vi "PAINEL DE TESTES 2808.vi"() -> ()   [LabVIEW 2019]
panel:
  in  "stop":bool
  out "ADDR NÃO COMPATÍVEL":bool
  in  "ME":bool
  in  "HMP":bool
  in  "SMP":bool
  out "TAM_P":bool
  out "POS_1":bool
  out "MAT":bool
  out "POS_2":bool
  out "COR_3":bool
  out "PDS":bool
  out "COR_2":bool
  out "PEE":bool
  out "POS_4":bool
  out "COR_1":bool
  out "POS_3":bool
  out "TAM_M":bool
  out "TAM_G":bool
  out "ADDR 100":bool
  out "ADDR 101":bool
  out "ADDR 011":bool
  out "ADDR 010":bool
  in  "ADDR ARRAY":bool[](array[boolean])
  out "INPUT ARRAYS":bool[](array[boolean])
  in  "time stamp":timestamp format="%<%X\n%x>T"
  # "UNIVERSIDADE FEDERAL DE SÃO JOÃO DEL-REI"
  # "CAMPUS ALTO PARAOPEBA - ENGENHARIA MECATRÔNICA\nLABORATÓRIO DE CONTROLE E AUTOMAÇÃO"
  # "PAINEL DE TESTES DO MÓDULO 2808"
  # "P1.0"
  # "P1.1"
  # "P1.2"
  # "D0"
  # "D1"
  # "D2"
  # "D3"
  # "D4"
  # "D5"
  # "D6"
  # "D7"
  # "ADDR 010"
  # "TAGS:\nPEE - PEÇA NA ENTRADA DA ESTEIRA\nMAT - MATERIAL DA PEÇA (T=METAL)\nCOR_1 - PEÇA DA COR 1\nCOR_2 - PEÇA DA COR 2\nCOR_3 - PEÇA DA COR 3\nTAM_G - PEÇA GRANDE\nTAM_M - PEÇA MÉDIA\nTAM_P - PEÇA PEQUENA\nPOS_1 - HASTE NA POSIÇÃO 1\nPOS_2 - HASTE NA POSIÇÃO 2\nPOS_3 - HASTE NA POSIÇÃO 3\nPOS_4 - HASTE NA POSIÇÃO 4\nPDS - PEÇA DEPOSITADA NO SLOT\n\nSMP - SENTIDO DO MOTOR DE PASSO\nHMP - HABILITA MOTOR DE PASSO\nME - MOTOR ESTEIRA"
  # "ADDR 011"
  # "ENCODER"
  # "ADDR 101"
  # "ADDR 100"
  # "TAM_G"
  # "TAM_P"
  # "TAM_M"
  # "SMP"
  # "POS_1"
  # "POS_2"
  # "POS_3"
  # "POS_4"
  # "PEE"
  # "MAT"
  # "COR_1,2,3"
  # "HMP"
  # "ME"
  # "PDS"
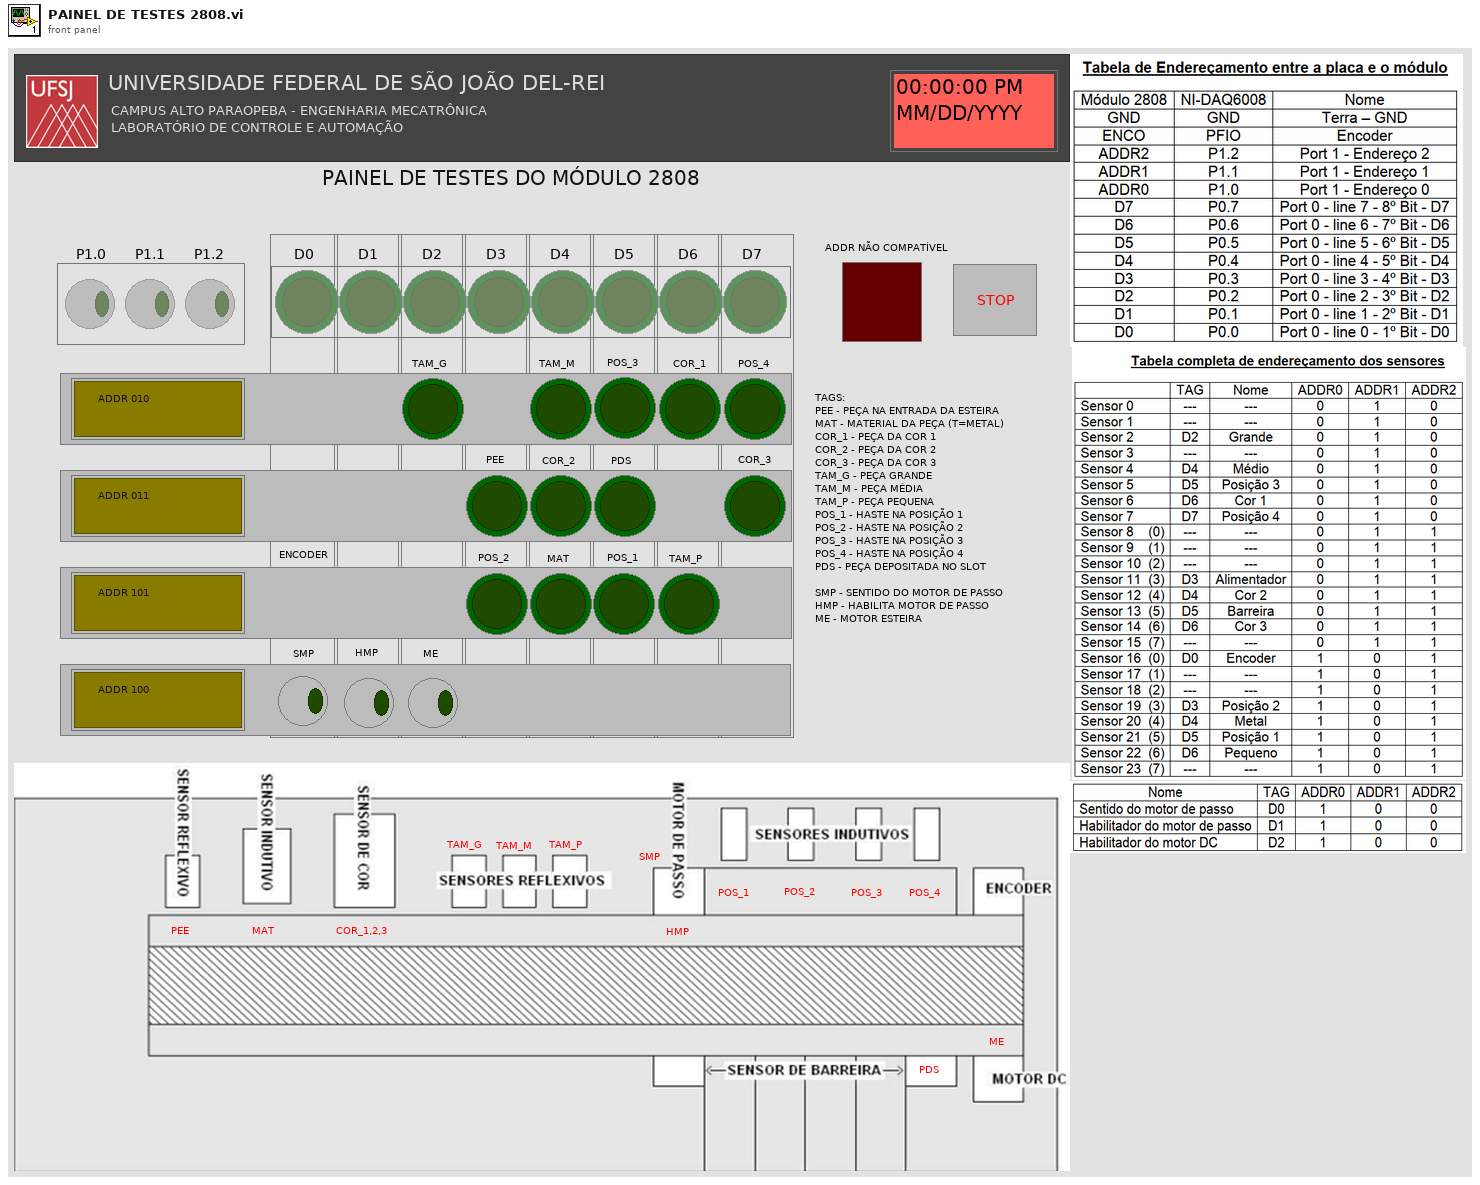
[diagram p1: front panel]
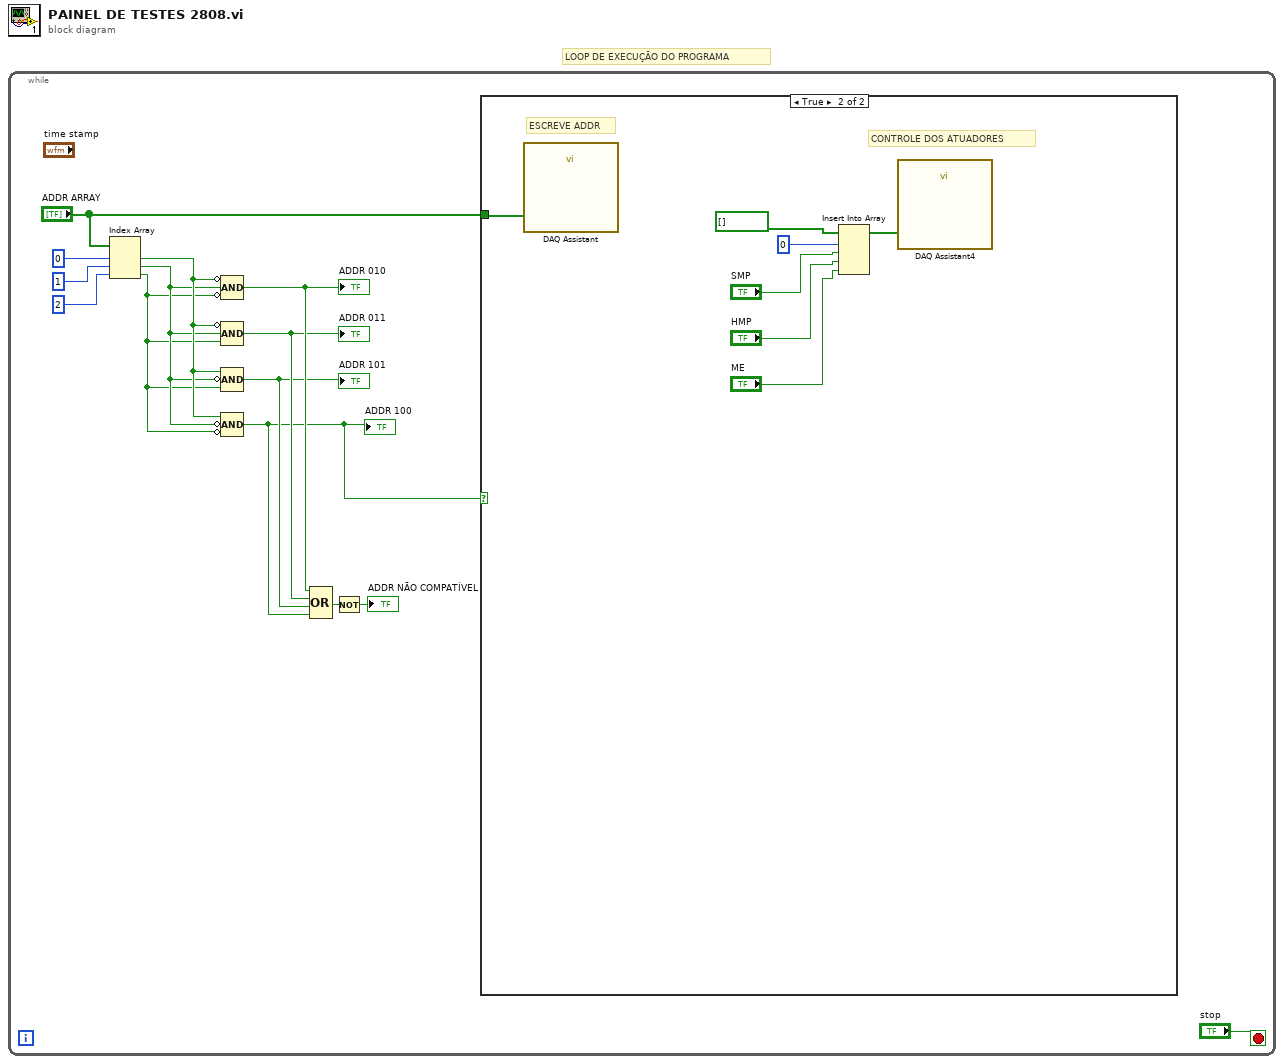
[diagram p0: block diagram]
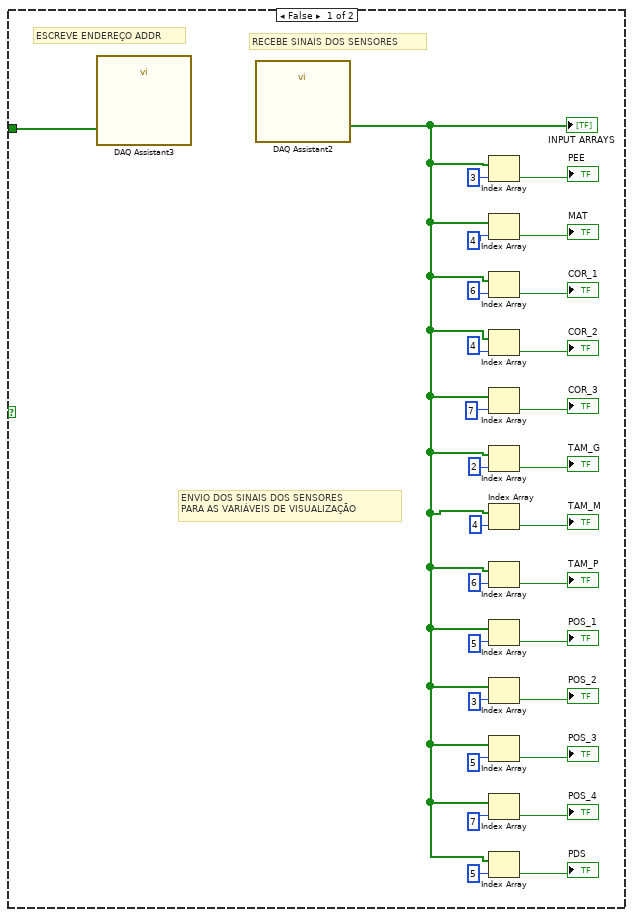
[diagram p2: hidden frame]
diagram:
  # "LOOP DE EXECUÇÃO DO PROGRAMA"
  n1 = while {
    stop <- "stop" stop-if-true
    n2 = Index Array(array="ADDR ARRAY", index #1=0 ("index"), index #2=1 ("index"), index #3=2 ("index")) -> (element #1=w10:bool, element #2=w9:bool, element #3=w8:bool)
    n3 = Compound Arithmetic op=AND(invert w10, w9, invert w8) -> (w7:bool)
    "ADDR 010" <- w7
    n4 = Compound Arithmetic op=AND(invert w10, w9, w8) -> (w6:bool)
    "ADDR 011" <- w6
    n5 = Compound Arithmetic op=AND(w10, invert w9, w8) -> (w5:bool)
    "ADDR 101" <- w5
    n6 = Compound Arithmetic op=AND(w10, invert w9, invert w8) -> (w4:bool)
    "ADDR 100" <- w4
    n7 = Compound Arithmetic op=OR(w7, w6, w5, w4) -> (w2:bool)
    n8 = Not(x=w2) -> (.not. x?=→"ADDR NÃO COMPATÍVEL":bool)
    n9 = case shown="True" w4 {
      tunnel: "ADDR ARRAY" -> [w42 w49]
      frame False {
        # "ENVIO DOS SINAIS DOS SENSORES\nPARA AS VARIÁVEIS DE VISUALIZAÇÃO"
        # "RECEBE SINAIS DOS SENSORES"
        # "ESCREVE ENDEREÇO ADDR"
        n10 = call "DAQ Assistant3"("data"=w42) -> ()  [unwired: 17 in, 2 out]
        n11 = call "DAQ Assistant2"() -> ("data"=w15:bool[])  [unwired: 17 in, 2 out]
        "INPUT ARRAYS" <- w15
        n12 = Index Array(array=w15, index=3) -> (element=→"PEE":bool)
        n13 = Index Array(array=w15, index=4) -> (element=→"MAT":bool)
        n14 = Index Array(array=w15, index=6) -> (element=→"COR_1":bool)
        n15 = Index Array(array=w15, index=4) -> (element=→"COR_2":bool)
        n16 = Index Array(array=w15, index=7) -> (element=→"COR_3":bool)
        n17 = Index Array(array=w15, index=2) -> (element=→"TAM_G":bool)
        n18 = Index Array(array=w15, index=4) -> (element=→"TAM_M":bool)
        n19 = Index Array(array=w15, index=6) -> (element=→"TAM_P":bool)
        n20 = Index Array(array=w15, index=5) -> (element=→"POS_1":bool)
        n21 = Index Array(array=w15, index=3) -> (element=→"POS_2":bool)
        n22 = Index Array(array=w15, index=5) -> (element=→"POS_3":bool)
        n23 = Index Array(array=w15, index=7) -> (element=→"POS_4":bool)
        n24 = Index Array(array=w15, index=5) -> (element=→"PDS":bool)
      }
      frame True {
        # "CONTROLE DOS ATUADORES"
        # "ESCREVE ADDR"
        n25 = call "DAQ Assistant"("data"=w49) -> ()  [unwired: 17 in, 2 out]
        n26 = Insert Into Array(array=bool[] [], index=0, new element #1="SMP", new element #2="HMP", new element #3="ME") -> (w43:bool[])
        n27 = call "DAQ Assistant4"("data"=w43) -> ()  [unwired: 17 in, 2 out]
      }
    }
  }
